vi "Send.vi"(8 "error in (no error)":errorcluster, 10 "Message":refnum<class "MSG.lvclass">, 11 "QueueMessenger in":refnum<class "QueueMessenger.lvclass">) -> (0 "error out":errorcluster, 3 "QueueMessenger out":refnum<class "QueueMessenger.lvclass">)   [LabVIEW 2011, in "Messenging.lvlib" / "QueueMessenger.lvclass"]
uses:
  QueueMessenger.lvclass
  Receiver/MGR (Receive type).lvclass
  TextVarientMessage/MSG.lvclass
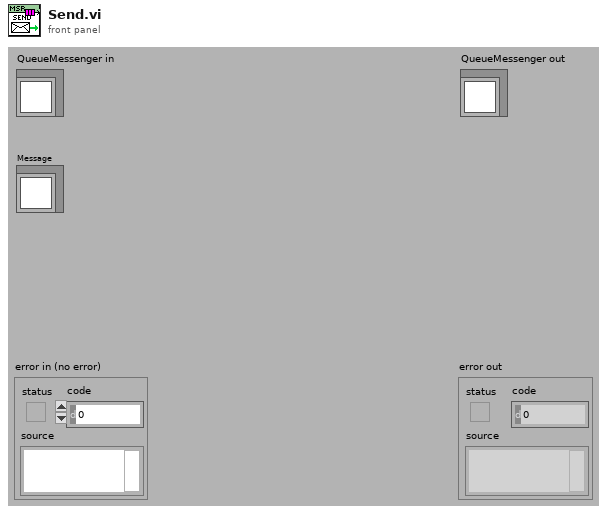
[diagram p1: front panel]
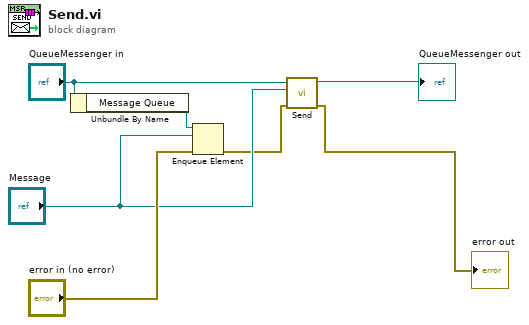
[diagram p0: block diagram]
diagram:
  n1 = Unbundle By Name("QueueMessenger in") -> ("Message Queue"=w7:refnum<queue>)
  n2 = Enqueue Element(queue=w7, element="Message", error in (no error)="error in (no error)") -> (error out=w2:errorcluster)  [unwired: 3 out]
  n3 = call-parent "Send.vi"("error in (no error)"=w2, "Message"="Message", "MSR Parent in"="QueueMessenger in") -> ("error out"=→"error out":errorcluster, "MSR Parent out"=→"QueueMessenger out":refnum<class "QueueMessenger.lvclass">)  [unwired: 7 out]
